vi "Util_App_DeleteTempDirectory.vi"(4 "error in":errorcluster, 7 "RootFolder":path) -> (0 "error out":errorcluster)   [LabVIEW 2023]
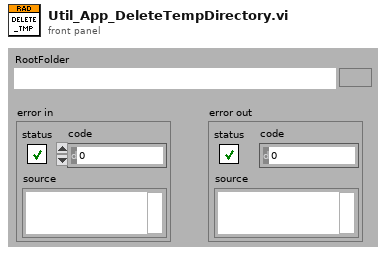
[diagram p1: front panel]
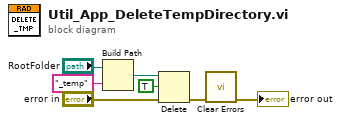
[diagram p0: block diagram]
diagram:
  n1 = Build Path(base path="RootFolder", name or relative path="_temp") -> (appended path=w5:path)
  n2 = Delete(path (use dialog)=w5, entire hierarchy (F)=TRUE, error in="error in") -> (error out=w3:errorcluster)  [unwired: 2 in, 2 out]
  n3 = call <vilib>:"Clear Errors.vi"("error in (no error)"=w3) -> ("error out"=→"error out":errorcluster)  [unwired: 5 in, 1 out]
